vi "Z_Stage.vi"(11 "Z-Coordinate":dbl) -> ()   [LabVIEW 2013]
panel:
  out "Current Z Position":sgl
  in  "MG17Motor 3":refnum<k7>(container)
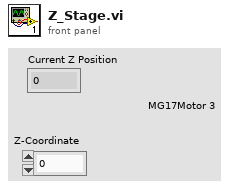
[diagram p1: front panel]
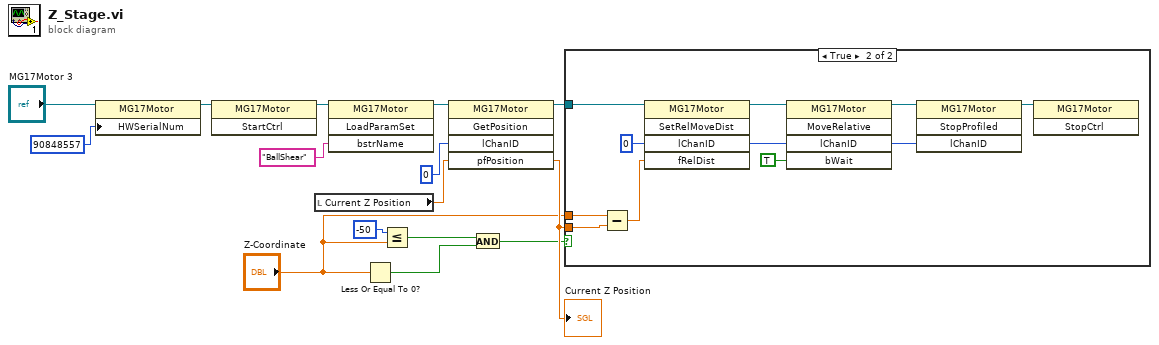
[diagram p0: block diagram]
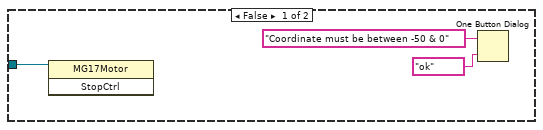
[diagram p2: hidden frame]
diagram:
  n1 = property class="MG17Motor"(reference="MG17Motor 3", "HWSerialNum"=90848557) -> (reference out=w14:refnum<k7>)  [unwired: 1 in, 1 out]
  n2 = invoke class="MG17Motor" method="StartCtrl"(reference=w14) -> (reference out=w2:refnum<k7>)  [unwired: 2 in, 2 out]
  n3 = local read "Current Z Position"() -> (w12:sgl)
  n4 = invoke class="MG17Motor" method="LoadParamSet"(reference=w2, "bstrName"="BallShear") -> (reference out=w1:refnum<k7>)  [unwired: 2 in, 3 out]
  n5 = Less Or Equal To 0?(x="Z-Coordinate") -> (x <= 0?=w4:bool)
  n6 = Less Or Equal?(x=-50, y="Z-Coordinate") -> (x <= y?=w6:bool)
  n7 = invoke class="MG17Motor" method="GetPosition"(reference=w1, "lChanID"=0, "pfPosition"=w12) -> (reference out=w9:refnum<k7>, "pfPosition"=w11:sgl)  [unwired: 2 in, 3 out]
  "Current Z Position" <- w11
  n8 = And(x=w6, y=w4) -> (x .and. y?=w10:bool)
  n9 = case shown="True" w10 {
    tunnel: "Z-Coordinate" -> [_ w19]
    tunnel: w11 -> [_ w20]
    tunnel: w9 -> [w18 w21]
    frame False {
      n10 = invoke class="MG17Motor" method="StopCtrl"(reference=w18) -> ()  [unwired: 2 in, 3 out]
      n11 = One Button Dialog(message="Coordinate must be between -50 & 0", button name ("OK")="ok") -> ()  [unwired: 1 out]
    }
    frame True {
      n12 = Subtract(x=w19, y=w20) -> (x-y=w22:dbl)
      n13 = invoke class="MG17Motor" method="SetRelMoveDist"(reference=w21, "lChanID"=0, "fRelDist"=w22) -> (reference out=w25:refnum<k7>, "lChanID"=w26:i32)  [unwired: 2 in, 3 out]
      n14 = invoke class="MG17Motor" method="MoveRelative"(reference=w25, "lChanID"=w26, "bWait"=TRUE) -> (reference out=w27:refnum<k7>, "lChanID"=w28:i32)  [unwired: 2 in, 3 out]
      n15 = invoke class="MG17Motor" method="StopProfiled"(reference=w27, "lChanID"=w28) -> (reference out=w29:refnum<k7>)  [unwired: 2 in, 3 out]
      n16 = invoke class="MG17Motor" method="StopCtrl"(reference=w29) -> ()  [unwired: 2 in, 3 out]
    }
  }
